vi "xy2ad.vi"(8 "Y (px)":dbl, 9 "X (px)":dbl, 11 "Astrometry":T1 {"LONGPOLE" format="%.1f"; "CRVAL" format="%_8g"; "CD" format="%_8g"; "NAXIS" format="%#.6g"}) -> (0 "DEC (°)":dbl format="%.6g", 1 "RA (°)":dbl format="%#.6g", 2 "DEC (HH:MM:SS)":dbl format="%<%H:%M:%S%3u>t", 3 "RA (HH:MM:SS.S)":dbl format="%<%H:%M:%S%1u>t")   [LabVIEW 2011]
uses:
  <vilib>/Analysis/Matrix/Numeric/Conversions/Array To Matrix - RA2.vi
  <vilib>/Analysis/baseanly.llb/Real Determinant.vi
  <vilib>/Analysis/Matrix/NI_Matrix.lvlib
  <vilib>/Analysis/NI_AALBase.lvlib
panel:
  out "eta":dbl format="%.6f"
  out "xsi":dbl format="%.6f"
  out "ydif":dbl
  out "xdif":dbl
  out "scale (°/px)":dbl
  out "scale (\"/px)":dbl
  out "teta":dbl
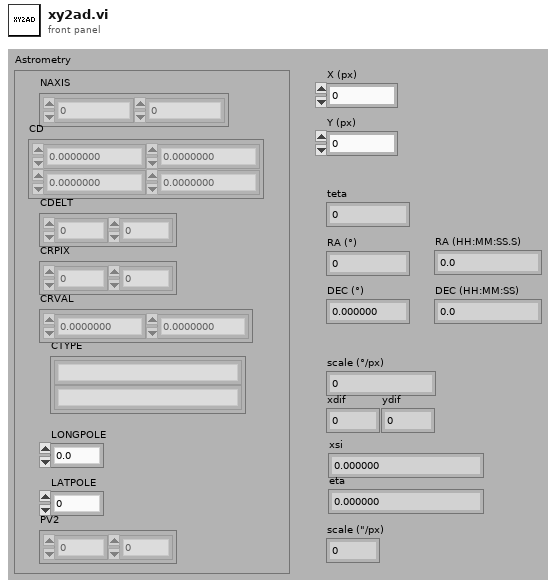
[diagram p1: front panel]
types:
  T1 = cluster{"NAXIS":dbl[], "CD":dbl[][], "CDELT":dbl[], "CRPIX":dbl[], "CTYPE":string[], "CRVAL":dbl[], "LONGPOLE":dbl, "LATPOLE":dbl, "PV2":dbl[]}
  T2 = typedef "NI_Matrix.lvlib/RealMatrix.ctl" = dbl[][]
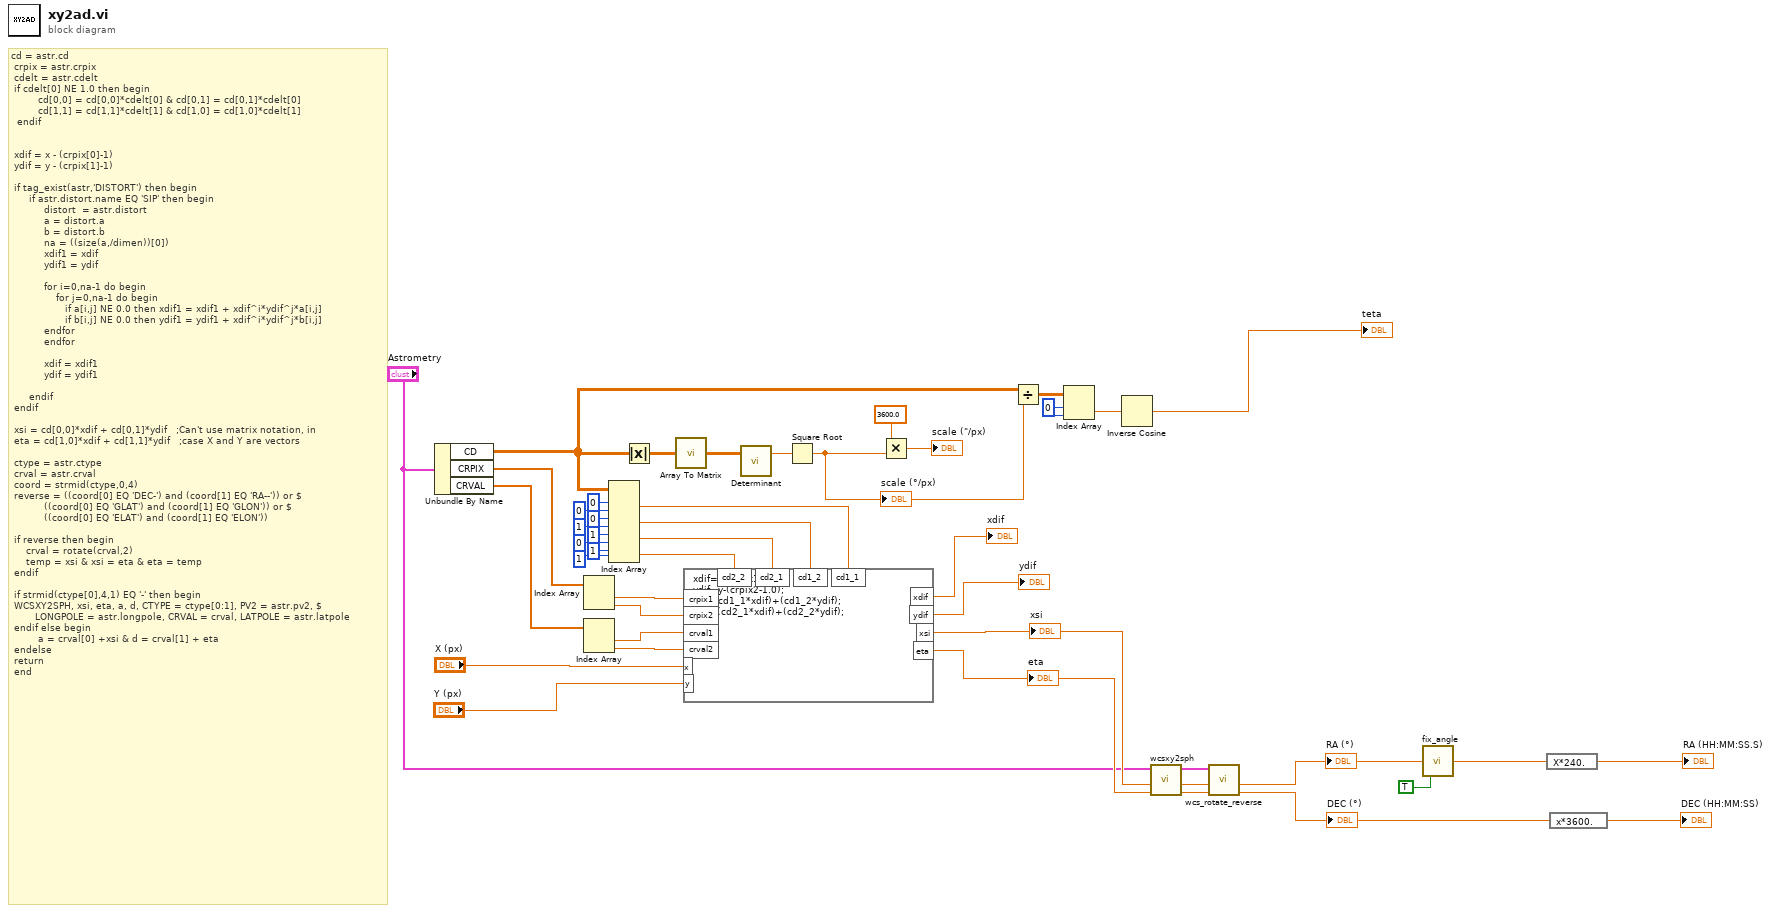
[diagram p0: block diagram]
diagram:
  w17 = 0 ("index (row)")
  # "cd = astr.cd\n crpix = astr.crpix\n cdelt = astr.cdelt\n if cdelt[0] NE 1.0 then begin \n         cd[0,0] = cd[0,0]*cdelt[0] & cd[0,1] = cd[0,1]*cdelt[0]\n         cd[1,1] = cd[1,1]*cdelt[1] & cd[1,0] = cd[1,0]*cdelt[1]\n  endif\n\n\n xdif = x - (crpix[0]-1)            \n ydif = y - (crpix[1]-1)\n \n if tag_exist(astr,'DISTORT') then begin\n      if astr.distort.name EQ 'SIP' then begin\n           distort  = astr.distort\n           a = distort.a\n           b = distort.b\n           na = ((size(a,/dimen))[0])\n           xdif1 = xdif\n           ydif1 = ydif\n           \n           for i=0,na-1 do begin\n               for j=0,na-1 do begin\n                  if a[i,j] NE 0.0 then xdif1 = xdif1 + xdif^i*ydif^j*a[i,j]            \n                  if b[i,j] NE 0.0 then ydif1 = ydif1 + xdif^i*ydif^j*b[i,j]\n           endfor\n           endfor\n\n           xdif = xdif1\n           ydif = ydif1\n           \n      endif\n endif\n\n xsi = cd[0,0]*xdif + cd[0,1]*ydif   ;Can't use matrix notation, in\n eta = cd[1,0]*xdif + cd[1,1]*ydif   ;case X and Y are vectors\n\n ctype = astr.ctype\n crval = astr.crval\n coord = strmid(ctype,0,4)\n reverse = ((coord[0] EQ 'DEC-') and (coord[1] EQ 'RA--')) or $\n           ((coord[0] EQ 'GLAT') and (coord[1] EQ 'GLON')) or $\n           ((coord[0] EQ 'ELAT') and (coord[1] EQ 'ELON'))\n\n if reverse then begin\n     crval = rotate(crval,2)\n     temp = xsi & xsi = eta & eta = temp\n endif\n\n if strmid(ctype[0],4,1) EQ '-' then begin\n WCSXY2SPH, xsi, eta, a, d, CTYPE = ctype[0:1], PV2 = astr.pv2, $\n        LONGPOLE = astr.longpole, CRVAL = crval, LATPOLE = astr.latpole\n endif else begin\n         a = crval[0] +xsi & d = crval[1] + eta\t\n endelse\n return\n end"
  n1 = Unbundle By Name("Astrometry") -> ("CD"=w21:dbl[][], "CRPIX"=w40:dbl[], "CRVAL"=w39:dbl[])
  n2 = Index Array(array=w40) -> (element #1=w38:dbl, element #2=w37:dbl)  [unwired: 2 in]
  n3 = Index Array(array=w39) -> (element #1=w36:dbl, element #2=w35:dbl)  [unwired: 2 in]
  n4 = Index Array(array=w21, index (row) #1=0 ("index (row)"), index (col) #1=0 ("disabled index (col)"), index (row) #2=0 ("index (row)"), index (col) #2=1 ("disabled index (col)"), index (row) #3=1 ("index (row)"), index (col) #3=0 ("disabled index (col)"), index (row) #4=1 ("index (row)"), index (col) #4=1 ("disabled index (col)")) -> (element #1=w26:dbl, element #2=w25:dbl, element #3=w24:dbl, element #4=w23:dbl)
  n5 = Absolute Value(x=w21) -> (abs(x)=w45:dbl[][])
  n6 = call-poly <vilib>:"Array To Matrix.vi"("Real 2D Array"=w45) -> ("Real Matrix"=w44:T2)
  n7 = formula code="xdif=x-(crpix1-1.0);\nydif=y-(crpix2-1.0);\nxsi=(cd1_1*xdif)+(cd1_2*ydif);\neta=(cd2_1*xdif)+(cd2_2*ydif);"("crval2"=w35, "crval1"=w36, "cd1_1"=w26, "cd1_2"=w25, "cd2_1"=w24, "cd2_2"=w23, "x"="X (px)", "y"="Y (px)", "crpix1"=w38, "crpix2"=w37) -> ("xdif"=→"xdif":dbl, "ydif"=→"ydif":dbl, "xsi"=w13:dbl, "eta"=w12:dbl)
  "xsi" <- w13
  "eta" <- w12
  n8 = call-poly <vilib>:"Determinant.vi"("Input Matrix"=w44) -> ("determinant"=w43:dbl)  [unwired: 1 in, 1 out]
  n9 = Square Root(x=w43) -> (sqrt(x)=w22:dbl)
  "scale (°/px)" <- w22
  n10 = Multiply(x=3600.0, y=w22) -> (x*y=→"scale (\"/px)":dbl)
  n11 = Divide(x=w21, y=w22) -> (x/y=w18:dbl[][])
  n12 = Index Array(array=w18, index (row)=w17, index (col)=w17) -> (element=w16:dbl)
  n13 = Inverse Cosine(1:w16) -> (0:→"teta":dbl)
  n14 = call "wcsxy2sph.vi"("Y"=w12, "X"=w13, "Astrometry"="Astrometry") -> ("lon"=w8:dbl, "lat"=w9:dbl, "Astrometry Dup"=w10:T1)  [unwired: 6 in]
  n15 = call "wcs_rotate_reverse.vi"("theta"=w8, "phi"=w9, "Astrometry"=w10) -> ("lat"=w6:dbl, "lon"=w2:dbl)  [unwired: 7 in]
  "RA (°)" <- w2
  "DEC (°)" <- w6
  n16 = call "fix_angle.vi"("±180 -> 0-360?"=TRUE, "Angle IN"=w2) -> ("Angle OUT"=w1:dbl)  [unwired: 3 in]
  n17 = expression code="X*240."(w1) -> (→"RA (HH:MM:SS.S)":dbl)
  n18 = expression code="x*3600."(w6) -> (→"DEC (HH:MM:SS)":dbl)
